vi "Start and End point of crosshair X axis.vi"(7 "For loop iteration":i32, 11 "Crosshair":T1={"Draw"=TRUE, "Target"={"x"=20.0, "y"=20.0}, "Size"={"x"=20.0, "y"=20.0}, "Angle"=1250067.0, "Color"=1250067, "Thickness"=20, "CrosshairLabel"=""} {"Thickness" max=0; "Target"."y" min=0.0 max=0.0; "Target"."x" min=0.0 max=0.0; "Angle" format="%#_13g"; "Size"."y" min=0.0 max=0.0; "Size"."x" min=0.0 max=0.0}) -> (1 "Scaling factor":i32, 2 "End point":cluster{i32, i32}, 3 "Start point":cluster{i32, i32})   [LabVIEW 2020]
uses:
  Controls/Crosshair type def.ctl
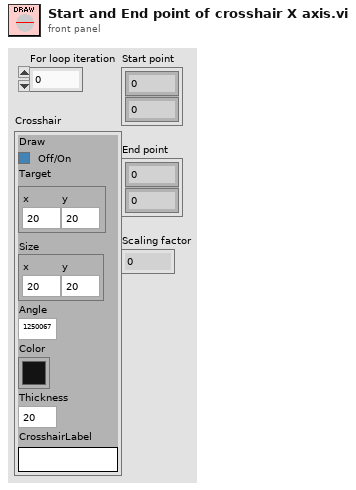
[diagram p1: front panel]
types:
  T1 = typedef "Crosshair type def.ctl" = cluster{"Draw":bool, "Target":cluster{"x":dbl, "y":dbl}, "Size":cluster{"x":dbl, "y":dbl}, "Angle":dbl, "Color":u32, "Thickness":u8, "CrosshairLabel":string}
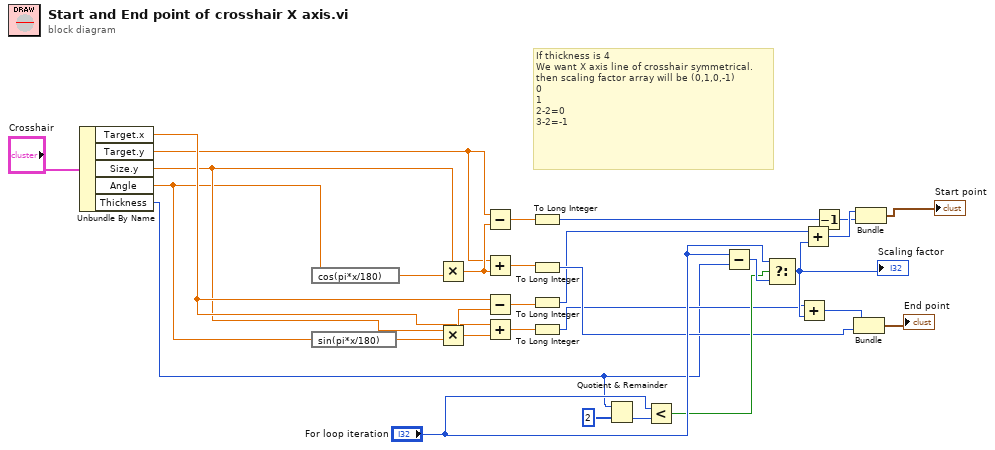
[diagram p0: block diagram]
diagram:
  # "If thickness is 4\nWe want X axis line of crosshair symmetrical.\nthen scaling factor array will be (0,1,0,-1)\n0\n1\n2-2=0\n3-2=-1"
  n1 = Unbundle By Name("Crosshair") -> ("Target.x"=w8:dbl, "Target.y"=w7:dbl, "Size.y"=w6:dbl, "Angle"=w5:dbl, "Thickness"=w4:u8)
  n2 = expression code="cos(pi*x/180)"(w5) -> (w17:dbl)
  n3 = expression code="sin(pi*x/180)"(w5) -> (w13:dbl)
  n4 = Multiply(x=w6, y=w17) -> (x*y=w18:dbl)
  n5 = Multiply(x=w6, y=w13) -> (x*y=w14:dbl)
  n6 = Subtract(x=w7, y=w18) -> (x-y=w20:dbl)
  n7 = Add(x=w7, y=w18) -> (x+y=w19:dbl)
  n8 = Subtract(x=w8, y=w14) -> (x-y=w15:dbl)
  n9 = Add(x=w8, y=w14) -> (x+y=w16:dbl)
  n10 = To Long Integer(number=w20) -> (32bit integer=w22:i32)
  n11 = To Long Integer(number=w19) -> (32bit integer=w23:i32)
  n12 = To Long Integer(number=w15) -> (32bit integer=w11:i32)
  n13 = To Long Integer(number=w16) -> (32bit integer=w10:i32)
  n14 = Quotient & Remainder(x=w4, y=2) -> (floor(x/y)=w25:i32)  [unwired: 1 out]
  n15 = Less?(x="For loop iteration", y=w25) -> (x < y?=w26:bool)
  n16 = Subtract(x="For loop iteration", y=w4) -> (x-y=w27:i32)
  n17 = Select(t="For loop iteration", s=w26, f=w27) -> (s? t:f=w29:i32)
  "Scaling factor" <- w29
  n18 = Add(x=w10, y=w29) -> (x+y=w21:i32)
  n19 = Add(x=w11, y=w29) -> (x+y=w2:i32)
  n20 = Decrement(x=w22) -> (x-1=w1:i32)
  n21 = Bundle(w21, w23) -> (→"End point":cluster{i32, i32})  [unwired: 1 in]
  n22 = Bundle(w2, w1) -> (→"Start point":cluster{i32, i32})  [unwired: 1 in]
